vi "Select Script_run_Re-enable Waveform Mode.vi"(7 "script name":string, 8 "Error In":errorcluster, 11 "Semiconductor Module Context":T1) -> (0 "Error Out":errorcluster)   [LabVIEW 2013]
uses:
  <vilib>/NI_TestStand_SemiconductorModule/NI_TestStand_Semiconductor_Module.lvlibp/PinMap/General/SemiconductorModuleContext.ctl
  <instrlib>/niHSDIO/niHSDIO.llb/niHSDIO_ctl Generation Mode Values (Ring).ctl
  <vilib>/NI_TestStand_SemiconductorModule/NI_TestStand_Semiconductor_Module.lvlibp
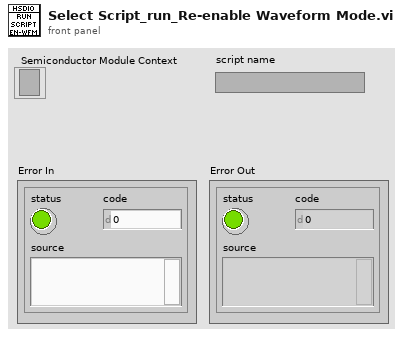
[diagram p1: front panel]
types:
  T1 = typedef "NI_TestStand_Semiconductor_Module.lvlibp/SemiconductorModuleContext.ctl" = refnum<k7>
  T2 = typedef "niHSDIO_ctl Generation Mode Values (Ring).ctl" = i32
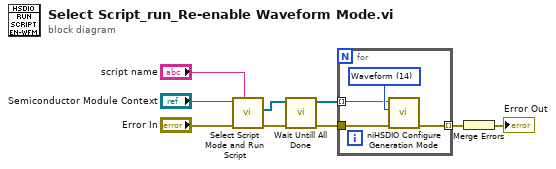
[diagram p0: block diagram]
diagram:
  n1 = call "Select Script Mode and Run Script.vi"("script name"="script name", "error in (no error)"="Error In", "Semiconductor Module Context"="Semiconductor Module Context") -> ("error out"=w6:errorcluster, "HSDIO GEN Sessions Out"=w1:refnum<k15>[])  [unwired: 6 in, 1 out]
  n2 = call "Wait Untill All Done.vi"("error in (no error)"=w6, "HSDIO Sessions In"=w1) -> ("error out"=w5:errorcluster, "HSDIO Sessions Out"=w4:refnum<k15>[])  [unwired: 8 in]
  n3 = for {
    tunnel: w5 -> [w12]
    tunnel: w4 -> [w11] mode=indexing
    tunnel: [w10] -> w3 mode=indexing
    w13 = T2 14 items=["Waveform"=14, "Scripted"=15] ("generation mode (waveform)")
    n4 = call <instrlib>:"niHSDIO Configure Generation Mode.vi"("error in (no error)"=w12, "generation mode (waveform)"=w13, "instrument handle"=w11) -> ("error out"=w10:errorcluster)  [unwired: 7 in, 1 out]
  }
  n5 = Merge Errors(w3) -> (→"Error Out":errorcluster)
